vi "IsString__slk_mt.vi"(7 "create enum configure":T1, 8 "error in (no error)":errorcluster, 11 "selection list":refnum<vi>[](array[refnum])) -> (0 "error out":errorcluster, 2 "position":cluster{"Left":i32, "Top":i32}, 3 "values":string[](array[string]), 4 "not?":bool)   [LabVIEW 2010]
uses:
  TypeDef/TypeDef_CreateEnumConfigure__slk_mt.ctl
  Library/Lazyboots Menu Tool.lvlib
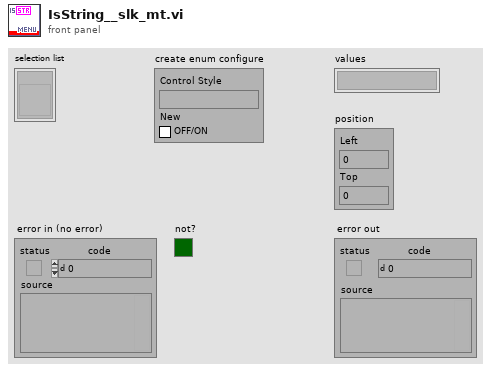
[diagram p1: front panel]
types:
  T1 = typedef "Lazyboots Menu Tool.lvlib/TypeDef_CreateEnumConfigure__slk_mt.ctl" = cluster{"Control Style":string, "New":bool}
  T2 = typedef "LVPositionTypeDef.ctl" = cluster{"Left":i32, "Top":i32}
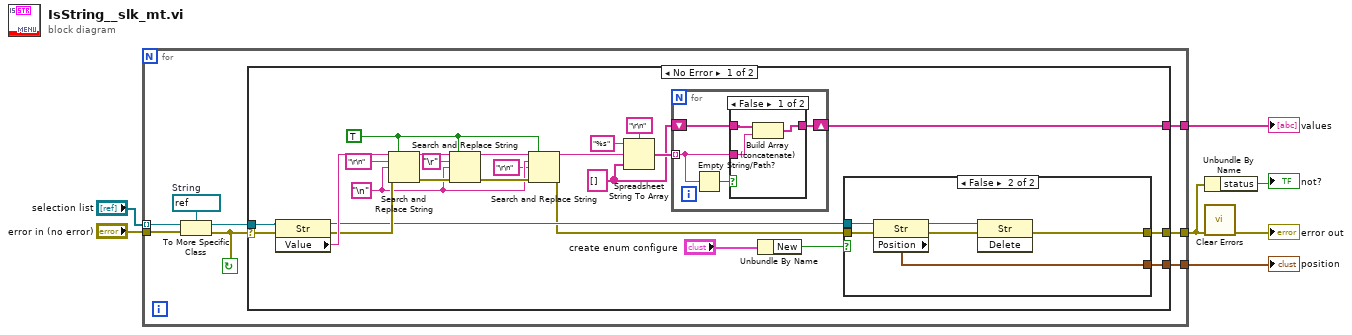
[diagram p0: block diagram]
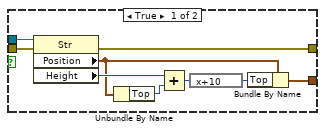
[diagram p2: hidden frame]
diagram:
  n1 = for {
    tunnel: "error in (no error)" -> [w15]
    tunnel: "selection list" -> [w13] mode=indexing
    tunnel: [w11] -> w4
    tunnel: [w9] -> w5
    tunnel: [w8] -> w1
    stop <- w12 continue-if-true
    w14 = refnum<vi> refnum  # String
    n2 = To More Specific Class(target class=w14, reference=w13, error in=w15) -> (specific class reference=w10:refnum<vi>, error out=w12:errorcluster)
    n3 = case shown="No Error" w12 {
      selector: w12 -> [w24 w64]
      tunnel: [w29 w64] -> w11
      tunnel: w10 -> [w25 _]
      tunnel: [w30 _] -> w9
      tunnel: [w23 _] -> w8
      frame No Error {
        w31 = string[] []
        w19 = "\n" ("search string")
        w16 = TRUE ("replace all? (F)")
        n4 = property class="Str"(reference=w25, error in=w24) -> (reference out=w28:refnum<vi>, error out=w36:errorcluster, "Value"=w37:string)
        n5 = Search and Replace String(replace all?=w16, input string=w37, search string="\r\n", replace string=w19, error in=w36) -> (result string=w38:string, error out=w35:errorcluster)  [unwired: 5 out]
        n6 = Search and Replace String(replace all?=w16, input string=w38, search string="\r", replace string=w19, error in=w35) -> (result string=w21:string, error out=w20:errorcluster)  [unwired: 5 out]
        n7 = Search and Replace String(replace all?=w16, input string=w21, search string=w19, replace string="\r\n" ("replace string (\"\")"), error in=w20) -> (result string=w22:string, error out=w17:errorcluster)  [unwired: 3 in, 2 out]
        n8 = Spreadsheet String To Array(delimiter (Tab)="\r\n" ("search string"), format string="%s", spreadsheet string=w22, array type (2D Dbl)=w31) -> (array=w32:string[])
        n9 = for {
          tunnel: w32 -> [w58] mode=indexing
          shift-right: [w56] -> w30
          shift-left: w31 -> [w57]
          n10 = Empty String/Path?(string/path=w58) -> (empty?=w59:bool)
          n11 = case shown="False" w59 {
            tunnel: w58 -> [w60 _]
            tunnel: w57 -> [w62 w63]
            tunnel: [w61 w63] -> w56
            frame False {
              n12 = Build Array (concatenate)(w62, w60) -> (w61:string[])
            }
            frame True {
            }
          }
        }
        n13 = Unbundle By Name("create enum configure") -> ("New"=w26:bool)
        n14 = case shown="False" w26 {
          tunnel: w17 -> [w46 w55]
          tunnel: [w44 w50] -> w29
          tunnel: w28 -> [w45 w54]
          tunnel: [w43 w53] -> w23
          frame True {
            n15 = property class="Str"(reference=w45, error in=w46) -> (error out=w44:errorcluster, "Position"=w42:T2, "Height"=w48:u32)  [unwired: 1 out]
            n16 = Unbundle By Name(w42) -> ("Top"=w47:i32)
            n17 = Add(x=w48, y=w47) -> (x+y=w49:u32)
            n18 = expression code="x+10"(w49) -> (w41:u32)
            n19 = Bundle By Name(cluster=w42, "Top"=w41) -> (w43:T2)
          }
          frame False {
            n20 = property class="Str"(reference=w54, error in=w55) -> (reference out=w51:refnum<vi>, error out=w52:errorcluster, "Position"=w53:T2)
            n21 = invoke class="Str" method="Delete"(reference=w51, error in=w52) -> (error out=w50:errorcluster)  [unwired: 1 in, 2 out]
          }
        }
      }
      frame Error {
      }
    }
  }
  "values" <- w5
  "position" <- w1
  n22 = Unbundle By Name(w4) -> ("status"=→"not?":bool)
  n23 = call <vilib>:"Clear Errors.vi"("error in (no error)"=w4) -> ("error out"=→"error out":errorcluster)  [unwired: 6 in]
